vi "Globals.vi"() -> ()   [LabVIEW 2015, in "TLB` Template.lvlib" / "AMC.lvlib"]
doc: "TLB Prime - Application Template 1.3.0.24\nNorm Kirchner, NI Systems Engineering - NI\nCopyright (c) 2014, NI"
uses:
  AMC.lvlib
panel:
  in  "Ack Message Name":string="AMC_Ack"
  in  "Default UDP Port":u16=54321
  in  "Dispatcher Process Name":string="AMC_Dispatch"
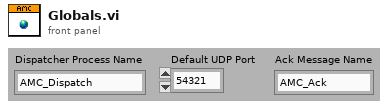
[diagram p1: front panel]
diagram:
